vi "_RT_CtrlLoop_MassAnalysing.vi"(6 "ExpVar in":refnum<class "ExpVar.lvclass">, 8 "error in (no error)":errorcluster, 11 "sig queue in":refnum<queue>) -> ()   [LabVIEW 2018]
uses:
  PublicSubVI/NewExpVar/ExpVar.lvclass
  <vilib>/Platform/TimedLoop/XDataNode/timing_clust.ctl
  <vilib>/Platform/TimedLoop/XDataNode/nitl_modes.ctl
  <vilib>/Platform/TimedLoop/XDataNode/wakeup.ctl
  PublicSubVI/Ctl/_ctl_RT_SysLog.ctl
  PublicSubVI/Ctl/_ctl_RT_FPGA_Function.ctl
  PublicSubVI/Ctl/_ctl_Integrated_Cmd.ctl
  <vilib>/Platform/TimedLoop/XDataNode/XDataNode.xnode
  <vilib>/Platform/TimedLoop/XDataNode/XDNodeRunTimeDep.lvlib
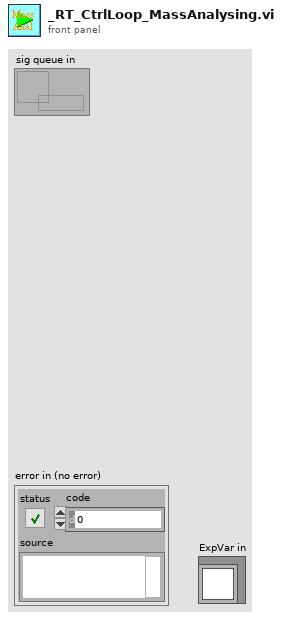
[diagram p1: front panel]
types:
  T1 = typedef "_ctl_RT_SysLog.ctl" = enum16{"None", "Initialize", "StartupRT", "StartupFPGA", "StartupAllocator", "GetMass", "SetWfmCode", "SetLaserCtrl", "SetTurboCtrl", "SetD999Ctrl", "Reconnecting...", "Interrupt", "StopRT"}
  T2 = typedef "_ctl_RT_FPGA_Function.ctl" = enum16{"Initialisation", "Execution", "Digital In"}
  T3 = typedef "XDNodeRunTimeDep.lvlib/timing_clust.ctl" = cluster{"Expected End [f-1]":u64, "Actual End [f-1]":u64, "Finished Late? [f-1]":bool, "Expected End [i-1]":u64, "Actual End [i-1]":u64, "Finished Late? [i-1]":bool, "Expected Start [i]":u64, "Actual Start [i]":u64, "Expected Start [f]":u64, "Actual Start [f]":u64, "Source Name":string, "Structure Name":string, "Period":i64, "Deadline":i64, "Offset":i64, "Start":i64, "Priority":i32, "Timeout":i32, "Mode":T4, "Wakeup Reason":T5, "Error":errorcluster, "Source Type":string, "Secondary Source Type":string, "Global End Time":u64, "Global Start Time":u64, "Frame Duration":u64, "Iteration Duration":u64, "Assigned CPU":i32, "I/O Scan Engine Mode":u32}
  T4 = typedef "XDNodeRunTimeDep.lvlib/nitl_modes.ctl" = enum32{"No Change", "Process missed periods, maintain original phase", "Discard missed periods, maintain original phase", "Process missed periods, ignore original phase", "Discard missed periods, ignore original phase"}
  T5 = typedef "XDNodeRunTimeDep.lvlib/wakeup.ctl" = enum32{"Normal", "Aborted", "Asynchronous wakeup", "Timing source error", "Timed loop error", "Timeout"}
  T6 = typedef "_ctl_Integrated_Cmd.ctl" = enum8{"Init", "Set", "Get", "Read", "Write", "Send", "Idle", "Startup", "Execution", "End", "Close"}
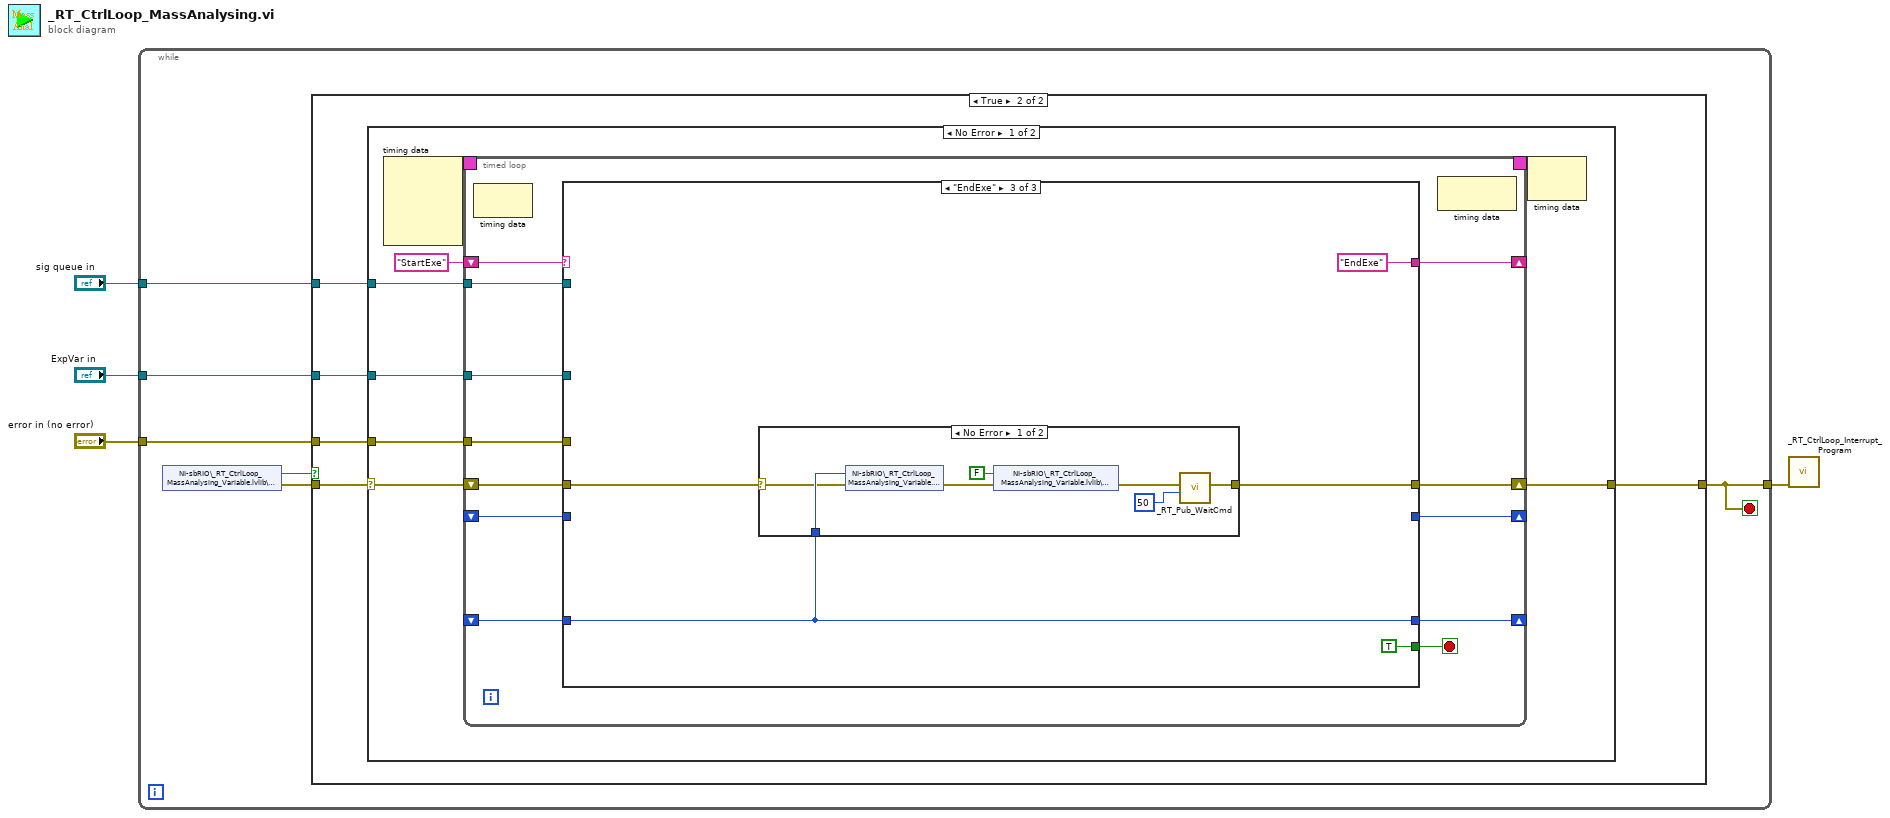
[diagram p0: block diagram]
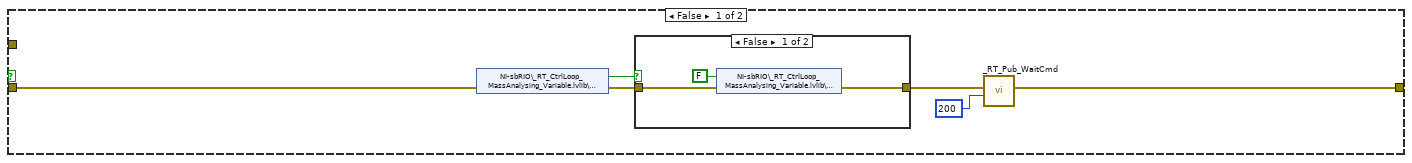
[diagram p2: hidden frame]
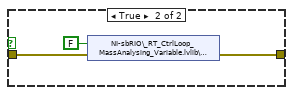
[diagram p3: hidden frame]
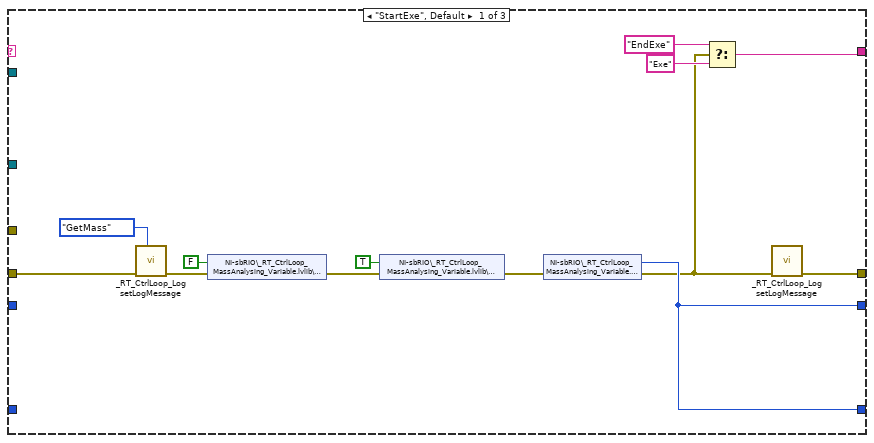
[diagram p4: hidden frame]
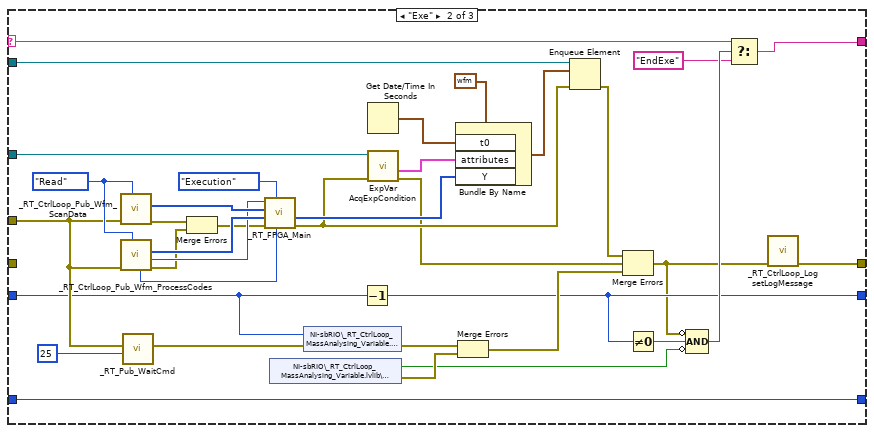
[diagram p5: hidden frame]
diagram:
  n1 = while {
    tunnel: "sig queue in" -> [w10]
    tunnel: "error in (no error)" -> [w9]
    tunnel: "ExpVar in" -> [w6]
    tunnel: [w5] -> w1
    stop <- w5 stop-if-true
    n2 = shared-variable "NI-sbRIO\\_RT_CtrlLoop_MassAnalysing_Variable.lvlib\\MassAnalExe"() -> (w8:bool, error out=w7:errorcluster)  [unwired: 1 in]
    n3 = case shown="True" w8 {
      tunnel: w7 -> [w16 w24]
      tunnel: w10 -> [_ w27]
      tunnel: [w12 w25] -> w5
      tunnel: w9 -> [_ w26]
      tunnel: w6 -> [_ w23]
      frame False {
        n4 = shared-variable "NI-sbRIO\\_RT_CtrlLoop_MassAnalysing_Variable.lvlib\\MassAnalPause"(error in=w16) -> (w15:bool, error out=w14:errorcluster)
        n5 = case shown="False" w15 {
          tunnel: w14 -> [w18 w21]
          tunnel: [w17 w20] -> w13
          frame False {
            n6 = shared-variable "NI-sbRIO\\_RT_CtrlLoop_MassAnalysing_Variable.lvlib\\MassAnalExe?"(FALSE ("MassAnalEnable"), error in=w18) -> (error out=w17:errorcluster)
          }
          frame True {
            n7 = shared-variable "NI-sbRIO\\_RT_CtrlLoop_MassAnalysing_Variable.lvlib\\MassAnalPause"(FALSE ("MassAnalPause"), error in=w21) -> (error out=w20:errorcluster)
          }
        }
        n8 = call "_RT_Pub_WaitCmd.vi"("milliseconds to wait"=u32 200, "error in (no error)"=w13) -> ("error out"=w12:errorcluster)  [unwired: 9 in]
      }
      frame True {
        n9 = case shown="No Error" w24 {
          selector: w24 -> [w30 w114]
          tunnel: w27 -> [w32 _]
          tunnel: w26 -> [w31 _]
          tunnel: [w29 w114] -> w25
          tunnel: w23 -> [w28 _]
          frame No Error {
            n10 = node-c288() -> (w35:T3)  [unwired: 4 in]
            n11 = timed-loop {
              timing: w35 -> [_]
              timing-out: [_] -> w34
              shift-right: [w46] -> _
              shift-left: "StartExe" -> [w47]
              shift-right: [w45] -> _
              shift-left: _ -> [w44]
              tunnel: w32 -> [w43]
              tunnel: w31 -> [w42]
              shift-right: [w41] -> _
              shift-left: _ -> [w40]
              tunnel: w28 -> [w37]
              shift-right: [w36] -> w29
              shift-left: w30 -> [w38]
              stop <- w39 stop-if-true
              n12 = node-c288() -> ()  [unwired: 1 in, 1 out]
              n13 = case shown="\"EndExe\"" w47 {
                selector: w47 -> [_ w95 _]
                tunnel: [w59 w94 "EndExe"] -> w46
                tunnel: [w60 w65 _] -> w45
                tunnel: w44 -> [_ w64 _]
                tunnel: w43 -> [_ w88 _]
                tunnel: w42 -> [_ w66 _]
                tunnel: [w49 w61 w98] -> w36
                tunnel: [_ _ TRUE ("MassAnalPause")] -> w39
                tunnel: [w60 w75 w99] -> w41
                tunnel: w40 -> [_ w75 w99]
                tunnel: w38 -> [w56 _ w97]
                tunnel: w37 -> [_ w70 _]
                frame "StartExe", Default {
                  n14 = call "_RT_CtrlLoop_Log setLogMessage.vi"("system type"=_ctl_RT_SysLog."GetMass", "error in"=w56) -> ("error out"=w55:errorcluster)  [unwired: 8 in, 1 out]
                  n15 = shared-variable "NI-sbRIO\\_RT_CtrlLoop_MassAnalysing_Variable.lvlib\\MassAnalExe"(FALSE ("MassAnalExe"), error in=w55) -> (error out=w52:errorcluster)
                  n16 = shared-variable "NI-sbRIO\\_RT_CtrlLoop_MassAnalysing_Variable.lvlib\\MassAnalExe?"(TRUE ("MassAnalEnable"), error in=w52) -> (error out=w51:errorcluster)
                  n17 = shared-variable "NI-sbRIO\\_RT_CtrlLoop_MassAnalysing_Variable.lvlib\\ExeTimes"(error in=w51) -> (w60:i32, error out=w50:errorcluster)
                  n18 = Select(t="EndExe" ("f"), s=w50, f="Exe") -> (s? t:f=w59:string)
                  n19 = call "_RT_CtrlLoop_Log setLogMessage.vi"("error in"=w50) -> ("error out"=w49:errorcluster)  [unwired: 9 in, 1 out]
                }
                frame "Exe" {
                  w83 = _ctl_Integrated_Cmd."Read" ("Enum")
                  n20 = call "_RT_CtrlLoop_Pub_Wfm_ScanData.vi"("Function"=w83, "error in (no error)"=w66) -> ("error out"=w82:errorcluster, "WFM_U64Arr out"=w91:u64[])  [unwired: 8 in]
                  n21 = call "_RT_CtrlLoop_Pub_Wfm_ProcessCodes.vi"("Function"=w83, "error in (no error)"=w66) -> ("error out"=w81:errorcluster, "SigLength out"=w89:i32, "EventCodes_U64Arr out"=w90:u64[], "DynamicTimeout"=w78:i32)  [unwired: 6 in]
                  n22 = call "_RT_Pub_WaitCmd.vi"("milliseconds to wait"=u32 25, "error in (no error)"=w66) -> ("error out"=w84:errorcluster)  [unwired: 9 in]
                  n23 = Merge Errors(w82, w81) -> (w80:errorcluster)
                  n24 = call "_RT_FPGA_Main.vi"("Timeout"=w78, "Function"=_ctl_RT_FPGA_Function."Execution", "Error in"=w80, "U64EventCodes"=w90, "U64ScanData_in"=w91, "Data_in"=w89) -> ("Error out"=w67:errorcluster, "SigData_out"=w69:i16[])  [unwired: 3 in, 1 out]
                  n25 = shared-variable "NI-sbRIO\\_RT_CtrlLoop_MassAnalysing_Variable.lvlib\\MassAnalPause"() -> (w71:bool, error out=w73:errorcluster)  [unwired: 1 in]
                  n26 = shared-variable "NI-sbRIO\\_RT_CtrlLoop_MassAnalysing_Variable.lvlib\\ExeTimes"(w64, error in=w84) -> (error out=w74:errorcluster)
                  n27 = Decrement(x=w64) -> (x-1=w65:i32)
                  n28 = Get Date/Time In Seconds() -> (seconds since 1Jan1904=w86:timestamp)
                  n29 = call-dynamic "ExpVar AcqExpCondition.vi"("error in (no error)"=w67, "ExpVar in"=w70) -> ("error out"=w63:errorcluster, "ExpCondition"=w68:cluster{"Label":string, "Value":variant}[])  [unwired: 7 in, 1 out]
                  n30 = Bundle By Name(cluster=waveform(i16) {"t0"=timestamp(0 s since 1904-01-01), "dt"=1.0, "Y"=[]} ("waveform"), "t0"=w86, "attributes"=w68, "Y"=w69) -> (w79:waveform(i16))
                  n31 = Merge Errors(w74, w73) -> (w72:errorcluster)
                  n32 = Enqueue Element(queue=w88, element=w79, error in (no error)=w67) -> (error out=w77:errorcluster)  [unwired: 1 in, 2 out]
                  n33 = Merge Errors(w77, w63, w72) -> (w62:errorcluster)
                  n34 = Not Equal To 0?(x=w65) -> (x != 0?=w76:bool)
                  n35 = Compound Arithmetic op=AND(invert w62, w76, invert w71) -> (w96:bool)
                  n36 = Select(t=w95, s=w96, f="EndExe") -> (s? t:f=w94:string)
                  n37 = call "_RT_CtrlLoop_Log setLogMessage.vi"("error in"=w62) -> ("error out"=w61:errorcluster)  [unwired: 9 in, 1 out]
                }
                frame "EndExe" {
                  n38 = case shown="No Error" w97 {
                    selector: w97 -> [w102 w109]
                    tunnel: w99 -> [w106 _]
                    tunnel: [w104 w109] -> w98
                    frame No Error {
                      n39 = shared-variable "NI-sbRIO\\_RT_CtrlLoop_MassAnalysing_Variable.lvlib\\ExeTimes"(w106, error in=w102) -> (error out=w107:errorcluster)
                      n40 = shared-variable "NI-sbRIO\\_RT_CtrlLoop_MassAnalysing_Variable.lvlib\\MassAnalExe?"(FALSE ("MassAnalEnable"), error in=w107) -> (error out=w105:errorcluster)
                      n41 = call "_RT_Pub_WaitCmd.vi"("milliseconds to wait"=u32 50, "error in (no error)"=w105) -> ("error out"=w104:errorcluster)  [unwired: 9 in]
                    }
                    frame Error {
                    }
                  }
                }
              }
              n42 = node-c288() -> ()  [unwired: 1 in, 1 out]
            }
            n43 = node-c288(w34) -> ()  [unwired: 1 out]
          }
          frame Error {
          }
        }
      }
    }
  }
  n44 = call "_RT_CtrlLoop_Interrupt_Program.vi"("error in (no error)"=w1) -> ()  [unwired: 10 in, 1 out]
